vi "诊断结果读取.vi"() -> ()   [LabVIEW 2018]
uses:
  <vilib>/Utility/NIReport.llb/Report Type.ctl
  <vilib>/Utility/NIReport.llb/Append Report Text (str wrap).vi
  <vilib>/Utility/NIReport.llb/NI_report.lvclass
  <vilib>/Utility/NIReport.llb/NI_ReportGenerationCore.lvlib
panel:
  in  "报表模板名称":string caption="报表模板名称（必须在“\\报表模板”目录下）"
  in  "保存报告":bool
  in  "内镜初步诊断报告":string
  out "日期：":string
  in  "报告医师":string
  out "图片文件":string
  in  "水平滑动杆 2":dbl(slide) scale=0.0..1171.0
  out "竖直滑动杆 2":cluster{dbl, dbl}(slide)={0.0, 3.1607515657620047}
  out "C扫图像 2":T1(plugin-control)
  in  "路径 3":path=path "E:/登陆系统重写/dist/predict"
  in  "路径":path=path "E:/登陆系统重写/待检测文件路径.txt"
  in  "路径 2":path=path "E:/登陆系统重写/保存文件路径.txt"
  in  "水平滑动杆":dbl(slide) scale=0.0..1171.0
  out "竖直滑动杆":cluster{dbl, dbl}(slide)={0.0, 3.1607515657620047}
  out "C扫图像":T1(plugin-control)
  in  "向前按钮":bool
  in  "确定按钮":bool
  in  "待检测文件":path
  in  "保存文件路径":path
  out "检测图片总数":i32
  out "当前图片名称":string
  in  "下一张":bool
  # "ME-NBI内镜图检测"
  # "图像显示"
  # "分割结果说明："
  # "的"
  # "低级别瘤变LGIN"
  # "肠化IM"
  # "的"
  # "炎症CG"
  # "的"
  # "图像文件夹选取"
  # "图像文件夹选取"
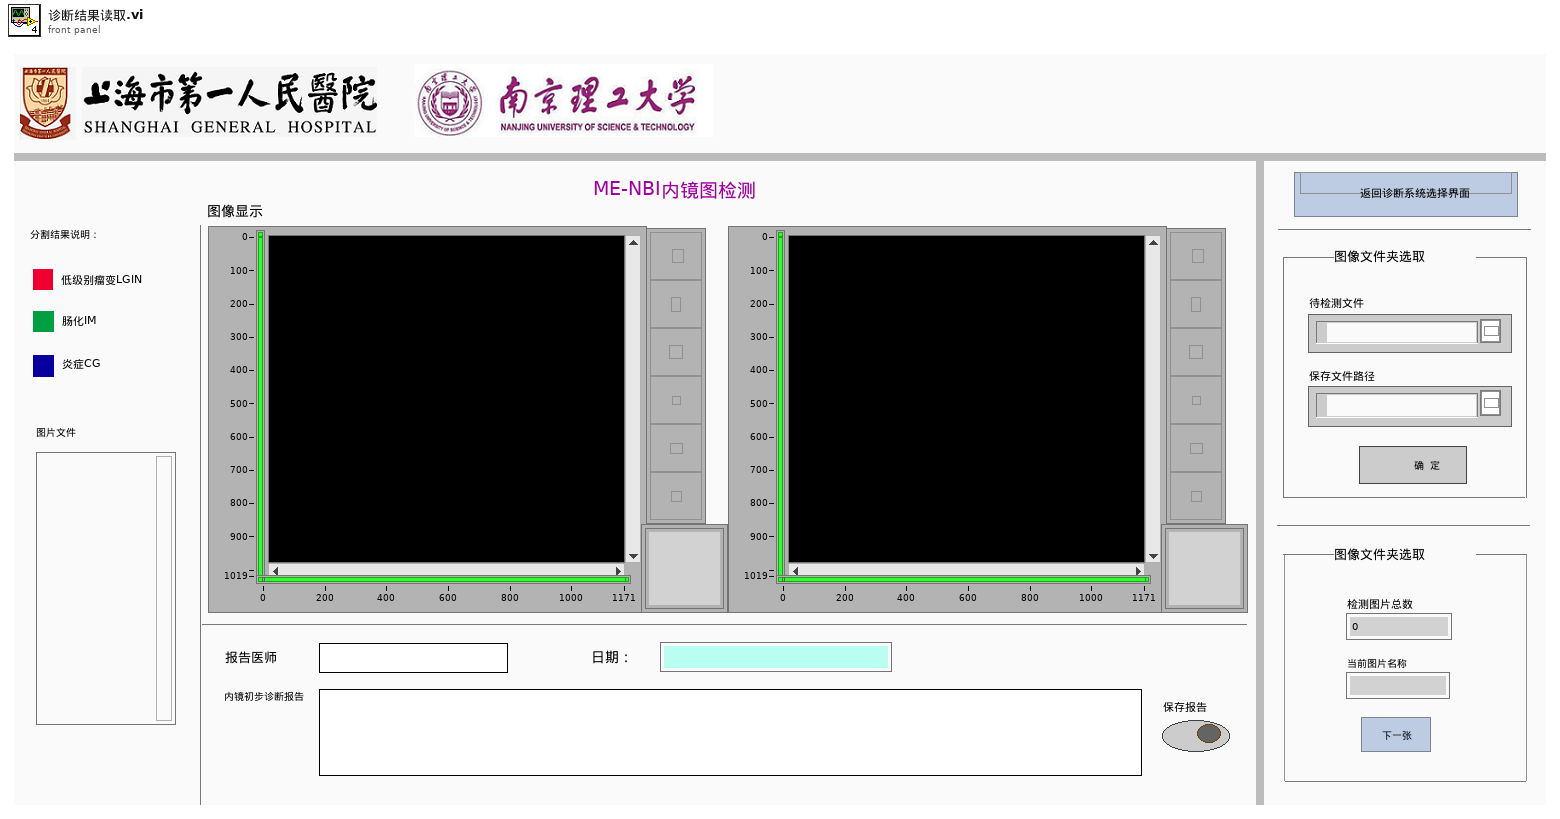
[diagram p1: front panel]
types:
  T1 = typedef "IMAQ Image.ctl" = refnum<image>
  T2 = typedef "Image Type" = u32
  T3 = enum16{"maximized", "minimized", "normal", "no change"}
  T4 = cluster{"position (Excel)":cluster{"row":i32, "column":i32}, "name (Excel)":string, "bookmark (Word)":string}
  T5 = typedef "NI_ReportGenerationCore.lvlib/Report Type.ctl" = enum16{"HTML", "Word", "Excel"}
  T6 = enum32{"Invalid", "Standard", "Closed", "Hidden", "Minimized", "Maximized"}
  T7 = enum16{"open", "replace", "create", "open or create", "replace or create", "replace or create with confirmation"}
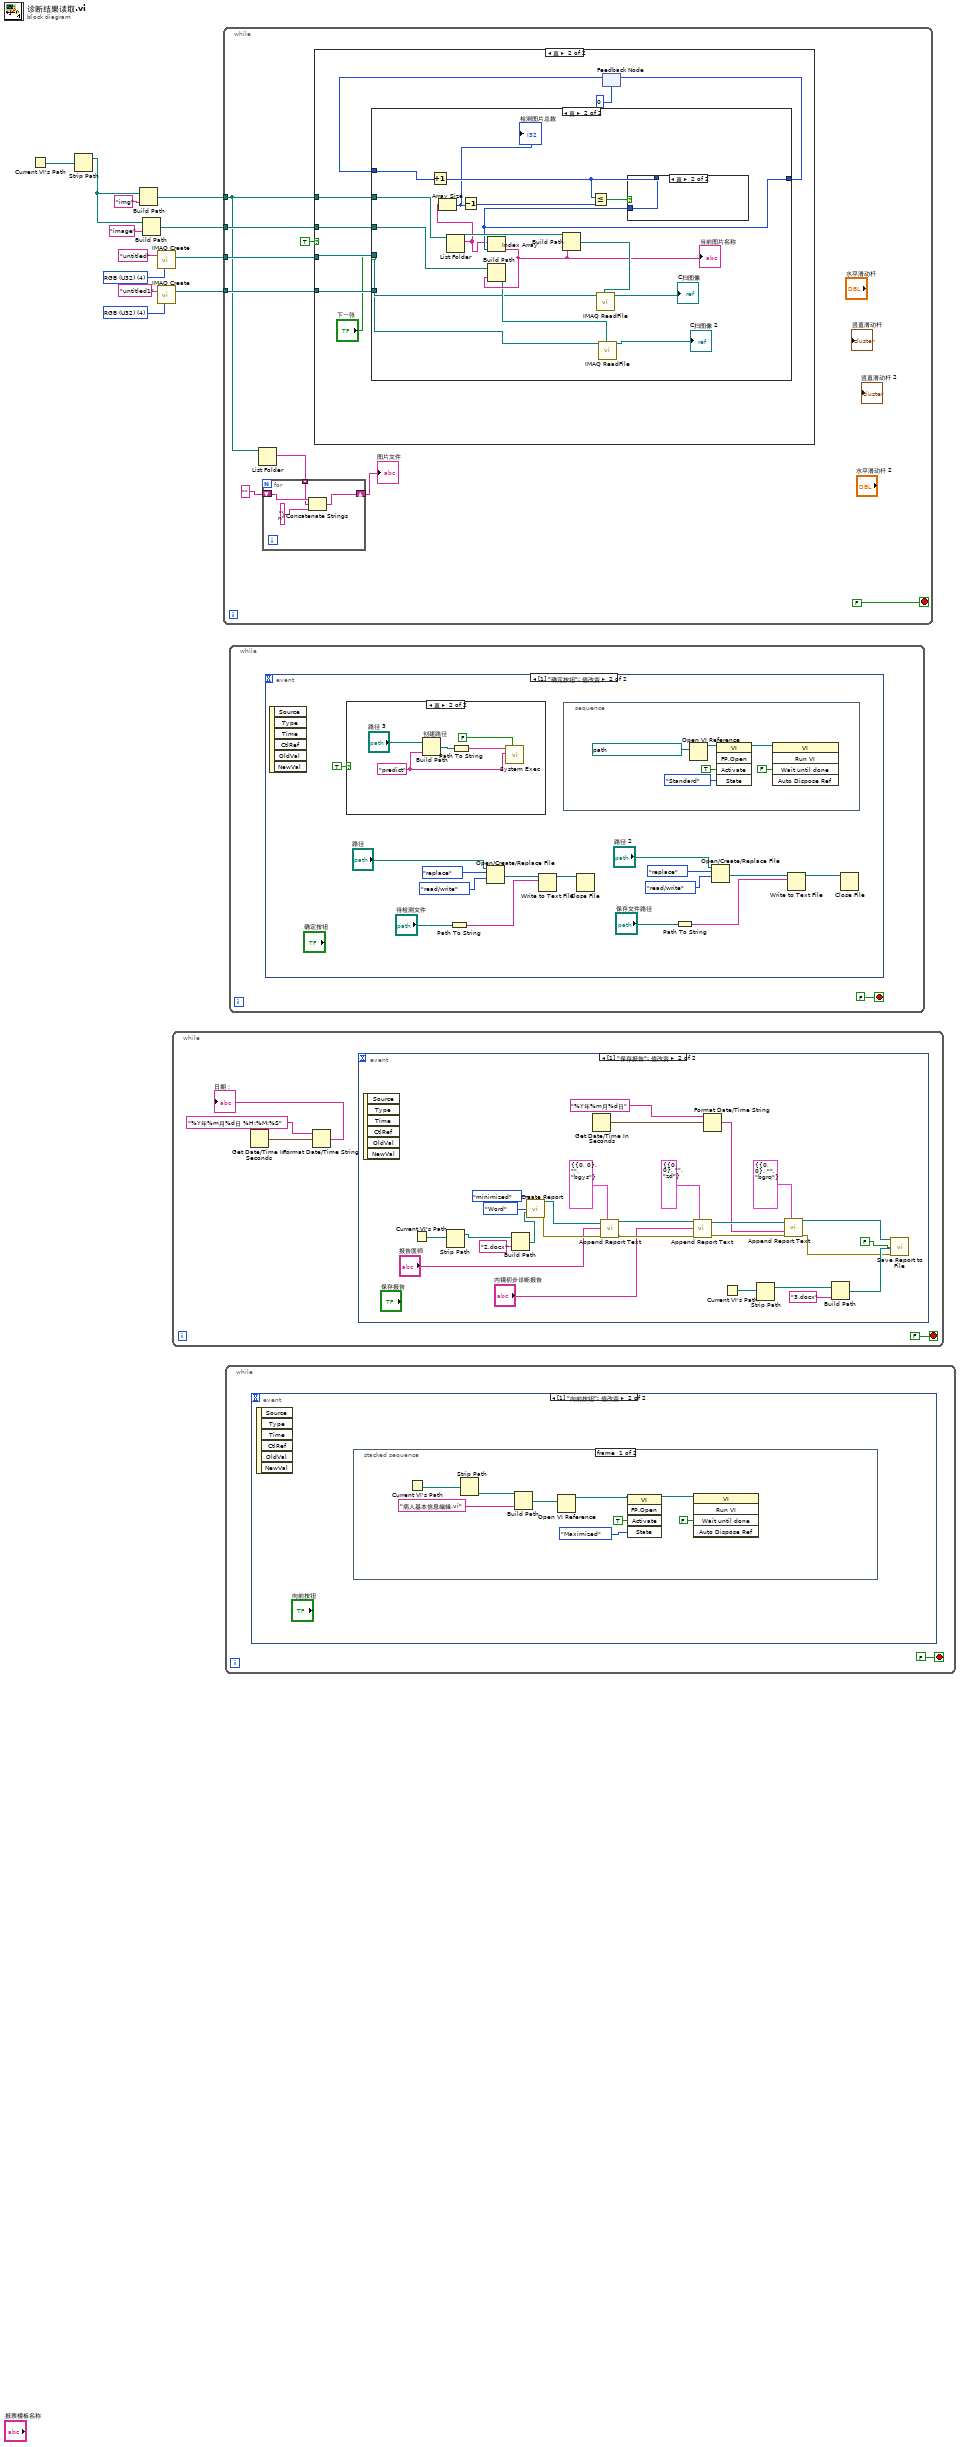
[diagram p0: block diagram]
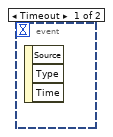
[diagram p2: hidden frame]
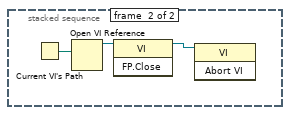
[diagram p3: hidden frame]
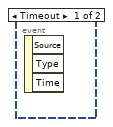
[diagram p4: hidden frame]
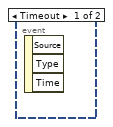
[diagram p5: hidden frame]
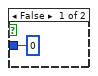
[diagram p9: hidden frame]
diagram:
  w10 = T2 4 items=["Grayscale (U8)", "Grayscale (I16)", "Grayscale (SGL)", "Complex (CSG)", "RGB (U32)", "HSL (U32)", "RGB (U64)", "Grayscale (U16)"] ("Image Type")
  w8 = T2 4 items=["Grayscale (U8)", "Grayscale (I16)", "Grayscale (SGL)", "Complex (CSG)", "RGB (U32)", "HSL (U32)", "RGB (U64)", "Grayscale (U16)"] ("Image Type")
  n1 = Current VI's Path() -> (path=w3:path)
  n2 = Strip Path(path=w3) -> (stripped path=w2:path)  [unwired: 1 out]
  n3 = Build Path(base path=w2, name or relative path="img" ("名称或相对路径")) -> (appended path=w1:path)
  n4 = Build Path(base path=w2, name or relative path="image" ("名称或相对路径")) -> (appended path=w6:path)
  n5 = call "IMAQ Create"("Image Name"="untitled", "Image Type"=w8) -> ("New Image"=w5:T1)  [unwired: 3 in, 1 out]
  n6 = call "IMAQ Create"("Image Name"="untitled1", "Image Type"=w10) -> ("New Image"=w4:T1)  [unwired: 3 in, 1 out]
  n7 = while {
    stop <- FALSE stop-if-true
    n8 = Get Date/Time In Seconds() -> (seconds since 1Jan1904=w14:timestamp)
    n9 = Format Date/Time String(time format string (%c)="%Y年%m月%d日 %H:%M:%S" ("时间格式字符串(%c)"), seconds (now)=w14) -> (date/time string=→"日期：":string)  [unwired: 1 in]
    n10 = event shown="[1] \"保存报告\": 值改变" {
      selector: _ -> [_ _]
      dyn-events: _ -> [_ _]
      timeout: _ -> [_ _]
      event Timeout {
        n11 = event-data() -> ()  [unwired: 1 in, 3 out]
      }
      event "保存报告": Value Change {
        n12 = event-data() -> ()  [unwired: 1 in, 6 out]
        n13 = Current VI's Path() -> (path=w42:path)
        n14 = Strip Path(path=w42) -> (stripped path=w41:path)  [unwired: 1 out]
        n15 = Build Path(base path=w41, name or relative path="2.docx" ("名称或相对路径")) -> (appended path=w43:path)
        n16 = call <vilib>:"Create Report.vi"("window state (normal)"=T3."minimized", "report type"=Report_Type."Word" ("Report Type"), "template (empty)"=w43) -> ("report out"=w40:refnum<class "NI_report.lvclass">, "error out"=w39:errorcluster)  [unwired: 11 in]
        n17 = Get Date/Time In Seconds() -> (seconds since 1Jan1904=w19:timestamp)
        n18 = call-poly <vilib>:"Append Report Text.vi"("report in"=w40, "MS Office parameters"=T4 {"position (Excel)"={"row"=0, "column"=0}, "name (Excel)"="", "bookmark (Word)"="bgys"}, "text"="报告医师", "error in (no error)"=w39) -> ("report out"=w35:refnum<class "NI_report.lvclass">, "error out"=w34:errorcluster)  [unwired: 8 in, 2 out]
        n19 = call-poly <vilib>:"Append Report Text.vi"("report in"=w35, "MS Office parameters"=T4 {"position (Excel)"={"row"=0, "column"=0}, "name (Excel)"="", "bookmark (Word)"="zd"}, "text"="内镜初步诊断报告", "error in (no error)"=w34) -> ("report out"=w31:refnum<class "NI_report.lvclass">, "error out"=w30:errorcluster)  [unwired: 8 in, 2 out]
        n20 = Format Date/Time String(time format string (%c)="%Y年%m月%d日" ("时间格式字符串(%c)"), seconds (now)=w19) -> (date/time string=w17:string)  [unwired: 1 in]
        n21 = Current VI's Path() -> (path=w38:path)
        n22 = Strip Path(path=w38) -> (stripped path=w37:path)  [unwired: 1 out]
        n23 = call-poly <vilib>:"Append Report Text.vi"("report in"=w31, "MS Office parameters"=T4 {"position (Excel)"={"row"=0, "column"=0}, "name (Excel)"="", "bookmark (Word)"="bgrq"}, "text"=w17, "error in (no error)"=w30) -> ("report out"=w29:refnum<class "NI_report.lvclass">, "error out"=w28:errorcluster)  [unwired: 8 in, 2 out]
        n24 = Build Path(base path=w37, name or relative path="3.docx" ("名称或相对路径")) -> (appended path=w36:path)
        n25 = call-dynamic "Save Report to File.vi"("report in"=w29, "report file path"=w36, "prompt to replace? (F)"=FALSE, "error in (no error)"=w28) -> ()  [unwired: 10 in, 2 out]
      }
    }
  }
  n26 = while {
    tunnel: w1 -> [w47]
    tunnel: w6 -> [w51]
    tunnel: w5 -> [w50]
    tunnel: w4 -> [w49]
    stop <- FALSE stop-if-true
    n27 = List Folder(path=w47) -> (filenames=w45:string[])  [unwired: 3 in, 3 out]
    n28 = for {
      shift-right: [w56] -> w44
      shift-left: "" -> [w55]
      tunnel: w45 -> [w53] mode=indexing
      n29 = Concatenate Strings(w55, w53, "\n" ("字符串")) -> (w56:string)
    }
    "图片文件" <- w44
    n30 = case shown="真" TRUE {
      tunnel: w47 -> [_ w63]
      tunnel: w51 -> [_ w62]
      tunnel: w50 -> [_ w61]
      tunnel: w49 -> [_ w60]
      frame False {
      }
      frame True {
        n31 = feedback #1(0) -> (w58:i32)
        n32 = case shown="真" "下一张" {
          tunnel: w63 -> [_ w78]
          tunnel: w62 -> [_ w77]
          tunnel: w61 -> [_ w76]
          tunnel: w60 -> [_ w75]
          tunnel: w58 -> [w65 w74]
          tunnel: [w65 w71] -> w57
          frame False {
          }
          frame True {
            n33 = Increment(x=w74) -> (x+1=w72:i32)
            n34 = List Folder ("罗列文件夹")(path=w78) -> (path out=w82:path, filenames=w66:string[])  [unwired: 3 in, 2 out]
            n35 = Array Size(array=w66) -> (size(s)=w69:i32)
            "检测图片总数" <- w69
            n36 = Decrement(x=w69) -> (x-1=w70:i32)
            n37 = Less Or Equal?(x=w72, y=w70) -> (x <= y?=w73:bool)
            n38 = case shown="真" w73 {
              tunnel: [0 w84] -> w71
              tunnel: w72 -> [_ w84]
              frame False {
              }
              frame True {
              }
            }
            n39 = Index Array(array=w66, index=w71) -> (element=w80:string)
            "当前图片名称" <- w80
            n40 = Build Path(base path=w77, name or relative path=w80) -> (appended path=w79:path)
            n41 = Build Path(base path=w82, name or relative path=w80) -> (appended path=w81:path)
            n42 = call "IMAQ ReadFile"("File Path"=w81, "Image"=w76) -> ("Image Out"=→"C扫图像":T1)  [unwired: 5 in, 4 out]
            n43 = call "IMAQ ReadFile"("File Path"=w79, "Image"=w75) -> ("Image Out"=→"C扫图像 2":T1)  [unwired: 5 in, 4 out]
          }
        }
        n44 = feedback-in #1(w57) -> ()
      }
    }
  }
  n45 = while {
    stop <- FALSE stop-if-true
    n46 = event shown="[1] \"向前按钮\": 值改变" {
      selector: _ -> [_ _]
      dyn-events: _ -> [_ _]
      timeout: _ -> [_ _]
      event Timeout {
        n47 = event-data() -> ()  [unwired: 1 in, 3 out]
      }
      event "向前按钮": Value Change {
        n48 = event-data() -> ()  [unwired: 1 in, 6 out]
        n49 = stacked-sequence {
          frame #0 {
            n50 = Current VI's Path() -> (path=w92:path)
            n51 = Strip Path(path=w92) -> (stripped path=w93:path)  [unwired: 1 out]
            n52 = Build Path(base path=w93, name or relative path="病人基本信息编辑.vi" ("名称或相对路径")) -> (appended path=w94:path)
            n53 = Open VI Reference(vi path=w94) -> (vi reference=w90:refnum<vi>)  [unwired: 5 in, 1 out]
            n54 = invoke class="VI" method="FP.Open"(reference=w90, "Activate"=TRUE ("激活？"), "State"=T6."Maximized" ("状态")) -> (reference out=w91:refnum<vi>)  [unwired: 2 in, 4 out]
            n55 = invoke class="VI" method="Run VI"(reference=w91, "Wait until done"=FALSE ("结束前等待")) -> ()  [unwired: 3 in, 5 out]
          }
          frame #1 {
            n56 = Current VI's Path() -> (path=w97:path)
            n57 = Open VI Reference(vi path=w97) -> (vi reference=w96:refnum<vi>)  [unwired: 5 in, 1 out]
            n58 = invoke class="VI" method="FP.Close"(reference=w96) -> (reference out=w95:refnum<vi>)  [unwired: 2 in, 2 out]
            n59 = invoke class="VI" method="Abort VI"(reference=w95) -> ()  [unwired: 2 in, 3 out]
          }
        }
      }
    }
  }
  n60 = while {
    stop <- FALSE stop-if-true
    n61 = event shown="[1] \"确定按钮\": 值改变" {
      selector: _ -> [_ _]
      dyn-events: _ -> [_ _]
      timeout: _ -> [_ _]
      event Timeout {
        n62 = event-data() -> ()  [unwired: 1 in, 3 out]
      }
      event "确定按钮": Value Change {
        n63 = event-data() -> ()  [unwired: 1 in, 6 out]
        n64 = case shown="真" TRUE {
          frame False {
          }
          frame True {
            w114 = "predict" ("名称或相对路径")
            n65 = Build Path "创建路径"(base path="路径 3", name or relative path=w114) -> (appended path=w116:path)
            n66 = Path To String(path=w116) -> (string=w117:string)
            n67 = call <vilib>:"System Exec.vi"("wait until completion? (T)"=FALSE, "standard input"=w114, "command line"=w117) -> ()  [unwired: 5 in, 4 out]
          }
        }
        n68 = Path To String(path="待检测文件") -> (string=w108:string)
        n69 = Open/Create/Replace File(file path (use dialog)="路径", operation (0:open)=T7."replace" ("操作(0:open)"), access (0:read/write)=enum16{"read/write", "read-only", "write-only"}."read/write" ("权限(0:read/write)")) -> (refnum out=w110:refnum<file>)  [unwired: 3 in, 2 out]
        n70 = Write to Text File(file (use dialog)=w110, text=w108) -> (refnum out=w109:refnum<file>)  [unwired: 2 in, 2 out]
        n71 = stacked-sequence {
          frame #0 {
            n72 = Open VI Reference(vi path=path "E:/登陆系统重写/进度条.vi" ("VI路径")) -> (vi reference=w124:refnum<vi>)  [unwired: 5 in, 1 out]
            n73 = invoke class="VI" method="FP.Open"(reference=w124, "Activate"=TRUE ("激活？"), "State"=T6."Standard" ("状态")) -> (reference out=w123:refnum<vi>)  [unwired: 2 in, 4 out]
            n74 = invoke class="VI" method="Run VI"(reference=w123, "Wait until done"=FALSE ("结束前等待")) -> ()  [unwired: 3 in, 5 out]
          }
        }
        n75 = Close File(refnum=w109) -> ()  [unwired: 1 in, 2 out]
        n76 = Path To String(path="保存文件路径") -> (string=w104:string)
        n77 = Open/Create/Replace File(file path (use dialog)="路径 2", operation (0:open)=T7."replace" ("操作(0:open)"), access (0:read/write)=enum16{"read/write", "read-only", "write-only"}."read/write" ("权限(0:read/write)")) -> (refnum out=w106:refnum<file>)  [unwired: 3 in, 2 out]
        n78 = Write to Text File(file (use dialog)=w106, text=w104) -> (refnum out=w105:refnum<file>)  [unwired: 2 in, 2 out]
        n79 = Close File(refnum=w105) -> ()  [unwired: 1 in, 2 out]
      }
    }
  }
